vi "PID Template Multi-Channel PID.vi"(0 "process variable":i16, 1 "reset?":bool, 12 "configuration":T1) -> (4 "output":i16, 10 "channel index":u16)   [LabVIEW 2017]
uses:
  <vilib>/Platform/TimedLoop/XDataNode/timing_clust.ctl
  <vilib>/Platform/TimedLoop/XDataNode/nitl_modes.ctl
  <vilib>/Platform/TimedLoop/XDataNode/wakeup.ctl
  <vilib>/rvi/DataTransferAndStorage/Container/Common/niFpgaContainerGetUniqueNameForEmu.vi
  <vilib>/rvi/DataTransferAndStorage/Container/Common/niFpgaContainerSetEmuInfo.vi
  <vilib>/rvi/eio/common/nirviEmuReportErrorAndStop.vi
  <vilib>/Platform/TimedLoop/XDataNode/XDataNode.xnode
  <vilib>/rvi/LocalResourceManager/LocalResourceManager.xnode
  <vilib>/Platform/TimedLoop/XDataNode/XDNodeRunTimeDep.lvlib
  <vilib>/addons/control/pid/NI_PID_FPGA.lvlib
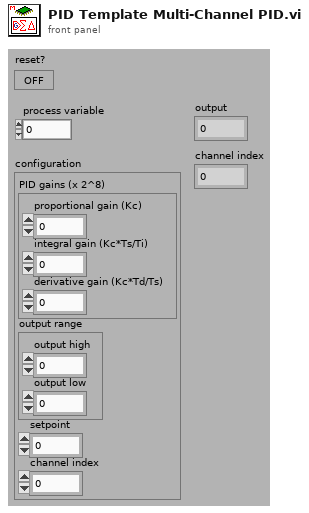
[diagram p1: front panel]
types:
  T1 = cluster{"PID gains (x 2^8)":cluster{"proportional gain (Kc)":i16, "integral gain (Kc*Ts/Ti)":i16, "derivative gain (Kc*Td/Ts)":i16}, "output range":cluster{"output high":i16, "output low":i16}, "setpoint":i16, "channel index":u16}
  T2 = typedef "XDNodeRunTimeDep.lvlib/timing_clust.ctl" = cluster{"Expected End [f-1]":u64, "Actual End [f-1]":u64, "Finished Late? [f-1]":bool, "Expected End [i-1]":u64, "Actual End [i-1]":u64, "Finished Late? [i-1]":bool, "Expected Start [i]":u64, "Actual Start [i]":u64, "Expected Start [f]":u64, "Actual Start [f]":u64, "Source Name":string, "Structure Name":string, "Period":i64, "Deadline":i64, "Offset":i64, "Start":i64, "Priority":i32, "Timeout":i32, "Mode":T3, "Wakeup Reason":T4, "Error":errorcluster, "Source Type":string, "Secondary Source Type":string, "Global End Time":u64, "Global Start Time":u64, "Frame Duration":u64, "Iteration Duration":u64, "Assigned CPU":i32, "I/O Scan Engine Mode":u32}
  T3 = typedef "XDNodeRunTimeDep.lvlib/nitl_modes.ctl" = enum32{"No Change", "Process missed periods, maintain original phase", "Discard missed periods, maintain original phase", "Process missed periods, ignore original phase", "Discard missed periods, ignore original phase"}
  T4 = typedef "XDNodeRunTimeDep.lvlib/wakeup.ctl" = enum32{"Normal", "Aborted", "Asynchronous wakeup", "Timing source error", "Timed loop error", "Timeout"}
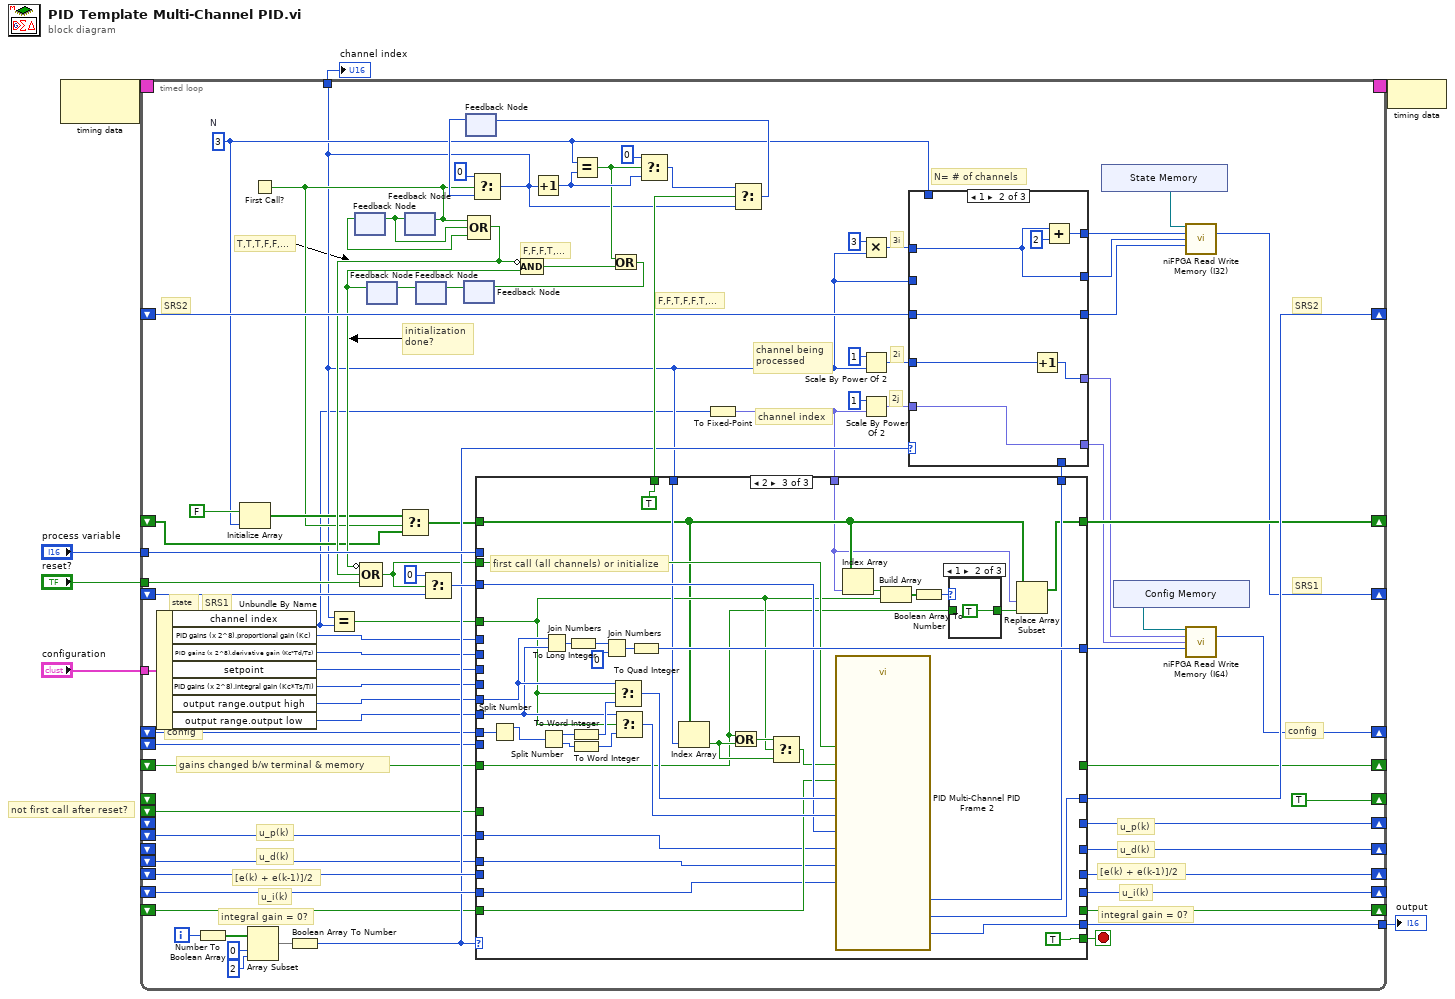
[diagram p0: block diagram]
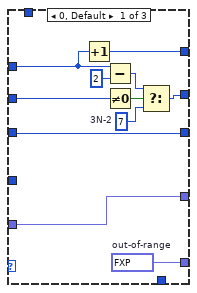
[diagram p2: hidden frame]
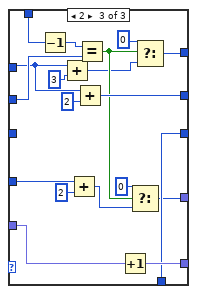
[diagram p3: hidden frame]
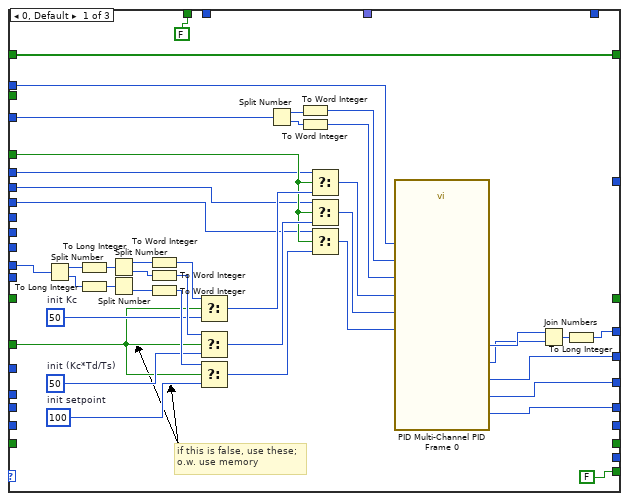
[diagram p4: hidden frame]
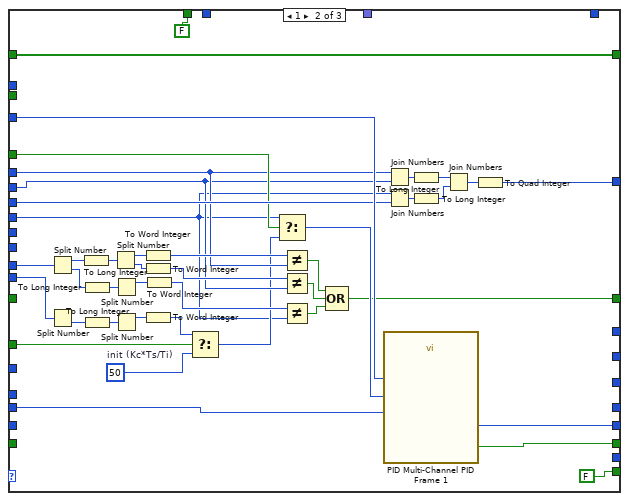
[diagram p5: hidden frame]
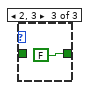
[diagram p7: hidden frame]
diagram:
  # "not first call after reset?"
  n1 = node-c288() -> (w7:T2)  [unwired: 1 out]
  n2 = timed-loop {
    timing: w7 -> [_]
    timing-out: [_] -> w6
    shift-right: [w89] -> _
    shift-left: _ -> [_]
    shift-right: [w90] -> _
    shift-left: _ -> [_]
    shift-right: [w88] -> _
    shift-left: _ -> [w58]
    tunnel: "process variable" -> [w87]
    shift-right: [w13] -> _
    shift-left: _ -> [w73]
    tunnel: "reset?" -> [w40]
    shift-right: [w80] -> _
    shift-left: _ -> [w79]
    shift-right: [w78] -> _
    shift-left: _ -> [w77]
    shift-right: [TRUE] -> _
    shift-right: [w12] -> _
    shift-left: _ -> [w59]
    shift-right: [w56] -> _
    shift-left: _ -> [w57]
    shift-left: _ -> [w60]
    shift-right: [w36] -> _
    shift-left: _ -> [w33]
    shift-left: _ -> [w47]
    shift-left: _ -> [w54]
    shift-left: _ -> [w53]
    shift-left: _ -> [_]
    tunnel: "configuration" -> [w39]
    tunnel: [w21] -> w2
    tunnel: [w37] -> w1
    shift-right: [w35] -> _
    shift-left: _ -> [w31]
    i -> [w71]
    stop <- w55 stop-if-true
    w28 = u16 3  # N
    # "2j"
    # "2i"
    # "3i"
    # "N= # of channels"
    # "F,F,T,F,F,T,..."
    # "F,F,F,T,..."
    # "T,T,T,F,F,..."
    # "config"
    # "channel index"
    # "channel being\nprocessed"
    # "SRS1"
    # "SRS2"
    # "SRS1"
    # "SRS2"
    # "config"
    # "state"
    # "u_i(k)"
    # "u_i(k)"
    # "initialization \ndone?"
    # "[e(k) + e(k-1)]/2"
    # "integral gain = 0?"
    # "u_d(k)"
    # "u_p(k)"
    # "[e(k) + e(k-1)]/2"
    # "u_p(k)"
    # "u_d(k)"
    # "integral gain = 0?"
    # "gains changed b/w terminal & memory"
    n3 = Unbundle By Name(w39) -> ("channel index"=w19:u16, "PID gains (x 2^8).proportional gain (Kc)"=w66:i16, "PID gains (x 2^8).derivative gain (Kc*Td/Ts)"=w65:i16, "setpoint"=w64:i16, "PID gains (x 2^8).integral gain (Kc*Ts/Ti)"=w63:i16, "output range.output high"=w62:i16, "output range.output low"=w61:i16)
    n4 = Number To Boolean Array(number=w71) -> (Boolean array=w76:bool[])
    n5 = Initialize Array(FALSE, w28) -> (w32:bool[])
    n6 = Array Subset(array=w76, index=0, length=2) -> (w72:bool[])
    n7 = First Call?() -> (First Call?: T/F=w29:bool)
    n8 = Boolean Array To Number(Boolean array=w72) -> (number=w68:u8)
    n9 = feedback #1() -> (w49:bool)  [unwired: 1 out]
    n10 = feedback #2() -> (w44:bool)  [unwired: 1 out]
    n11 = Select(t=w32, s=w29, f=w31) -> (s? t:f=w30:bool[])
    n12 = feedback-in #3(w29) -> ()
    n13 = feedback #3() -> (w50:bool)  [unwired: 1 out]
    n14 = feedback-in #1(w50) -> ()
    n15 = feedback #4() -> (w45:bool)  [unwired: 1 out]
    n16 = feedback-in #2(w45) -> ()
    n17 = feedback #5() -> (w43:bool)  [unwired: 1 out]
    n18 = feedback-in #4(w43) -> ()
    n19 = feedback #6() -> (w51:u16)  [unwired: 1 out]
    n20 = Compound Arithmetic op=OR(w29, w50, w49) -> (w48:bool)
    n21 = Compound Arithmetic op=OR(invert w44, w48, w40) -> (w41:bool)
    n22 = Select(t=0 ("Data"), s=w41, f=w73) -> (s? t:f=w69:i32)
    n23 = Select(t=u16 0, s=w29, f=w51) -> (s? t:f=w21:u16)
    n24 = Equal?(x=w21, y=w19) -> (x = y?=w67:bool)
    n25 = Compound Arithmetic op=AND(invert w48, w44) -> (w83:bool)
    n26 = Increment(x=w21) -> (x+1=w84:u16)
    n27 = Equal?(x=w28, y=w84) -> (x = y?=w82:bool)
    n28 = Or(x=w82, y=w83) -> (x .or. y?=w42:bool)
    n29 = feedback-in #5(w42) -> ()
    n30 = Select(t=u16 0, s=w82, f=w84) -> (s? t:f=w85:u16)
    n31 = To Fixed-Point(number=w19) -> (fixed-point=w18:fxp<+,17,17>)  [unwired: 1 out]
    n32 = case shown="2" w68 {
      tunnel: [w166 _ _] -> w90
      tunnel: [w167 _ _] -> w89
      tunnel: [_ w209 _] -> w88
      tunnel: w54 -> [_ _ w213]
      tunnel: w53 -> [_ _ w212]
      tunnel: w87 -> [w164 _ _]
      tunnel: [FALSE FALSE TRUE] -> w81
      tunnel: [w165 _ _] -> w80
      tunnel: w79 -> [_ w184 _]
      tunnel: [_ w208 _] -> w78
      tunnel: w77 -> [_ _ w211]
      tunnel: w69 -> [w161 w207 w236]
      tunnel: [w157 _ w233] -> w56
      tunnel: [_ w175 _] -> w36
      tunnel: w67 -> [w135 w176 w221]
      tunnel: w66 -> [w134 w174 _]
      tunnel: w65 -> [w133 w173 _]
      tunnel: w64 -> [w132 w183 _]
      tunnel: w63 -> [_ w170 _]
      tunnel: w62 -> [_ _ w238]
      tunnel: w61 -> [_ _ w237]
      tunnel: w60 -> [_ w186 _]
      tunnel: w47 -> [w137 w188 _]
      tunnel: w59 -> [w136 w189 w247]
      tunnel: [_ w179 w240] -> w9
      tunnel: w58 -> [_ _ w232]
      tunnel: w33 -> [_ _ w215]
      tunnel: [FALSE FALSE TRUE] -> w55
      tunnel: w41 -> [_ _ w229]
      tunnel: [_ _ w231] -> w38
      tunnel: [_ _ w230] -> w37
      tunnel: w30 -> [w128 w169 w218]
      tunnel: w21 -> [_ _ w226]
      tunnel: w18 -> [_ _ w217]
      tunnel: [w128 w169 w225] -> w35
      frame 0, Default {
        w141 = i16 100  # init setpoint
        w143 = i16 50  # init Kc
        w142 = i16 50  # init (Kc*Td/Ts)
        # "if this is false, use these; \no.w. use memory"
        n33 = Split Number(x=w136) -> (hi(x)=w144:u32, lo(x)=w145:u32)
        n34 = To Long Integer(number=w144) -> (32bit integer=w155:i32)
        n35 = To Long Integer(number=w145) -> (32bit integer=w156:i32)
        n36 = Split Number(x=w155) -> (hi(x)=w146:u16, lo(x)=w148:u16)
        n37 = Split Number(x=w156) -> (lo(x)=w150:u16)  [unwired: 1 out]
        n38 = To Word Integer(number=w146) -> (16bit integer=w147:i16)
        n39 = To Word Integer(number=w148) -> (16bit integer=w149:i16)
        n40 = To Word Integer(number=w150) -> (16bit integer=w151:i16)
        n41 = Select(t=w147, s=w137, f=w143) -> (s? t:f=w152:i16)
        n42 = Select(t=w149, s=w137, f=w142) -> (s? t:f=w153:i16)
        n43 = Select(t=w151, s=w137, f=w141) -> (s? t:f=w154:i16)
        n44 = Split Number(x=w161) -> (hi(x)=w162:u16, lo(x)=w163:u16)
        n45 = To Word Integer(number=w162) -> (16bit integer=w160:i16)
        n46 = To Word Integer(number=w163) -> (16bit integer=w159:i16)
        n47 = Select(t=w134, s=w135, f=w152) -> (s? t:f=w140:i16)
        n48 = Select(t=w133, s=w135, f=w153) -> (s? t:f=w139:i16)
        n49 = Select(t=w132, s=w135, f=w154) -> (s? t:f=w138:i16)
        n50 = call <vilib>:"PID Multi-Channel PID Frame 0.vi"("setpoint"=w138, "proportional gain (Kc) (k)"=w140, "derivative gain (Kc*Td/Ts) (k)"=w139, "PV(k)"=w164, "e(k-1)"=w159, "PV(k-1)"=w160) -> ("[e(k)+e(k-1)]/2"=w165:i16, "PV(k)"=w131:i16, "e(k)"=w130:i16, "u_p(k)"=w167:i32, "u_d(k)"=w166:i32)  [unwired: 5 out]
        n51 = Join Numbers(hi=w131, lo=w130) -> ((hi.lo)=w158:u32)
        n52 = To Long Integer(number=w158) -> (32bit integer=w157:i32)
      }
      frame 1 {
        w187 = i16 50  # init (Kc*Ts/Ti)
        n53 = Split Number(x=w189) -> (hi(x)=w194:u32, lo(x)=w198:u32)
        n54 = Split Number(x=w186) -> (lo(x)=w191:u32)  [unwired: 1 out]
        n55 = To Long Integer(number=w194) -> (32bit integer=w195:i32)
        n56 = To Long Integer(number=w198) -> (32bit integer=w197:i32)
        n57 = To Long Integer(number=w191) -> (32bit integer=w192:i32)
        n58 = Split Number(x=w195) -> (hi(x)=w196:u16, lo(x)=w199:u16)
        n59 = Split Number(x=w197) -> (hi(x)=w200:u16)  [unwired: 1 out]
        n60 = Split Number(x=w192) -> (hi(x)=w193:u16)  [unwired: 1 out]
        n61 = To Word Integer(number=w196) -> (16bit integer=w201:i16)
        n62 = To Word Integer(number=w199) -> (16bit integer=w202:i16)
        n63 = To Word Integer(number=w193) -> (16bit integer=w185:i16)
        n64 = To Word Integer(number=w200) -> (16bit integer=w203:i16)
        n65 = Select(t=w185, s=w188, f=w187) -> (s? t:f=w172:i16)
        n66 = Select(t=w170, s=w176, f=w172) -> (s? t:f=w190:i16)
        n67 = Not Equal?(x=w201, y=w174) -> (x != y?=w204:bool)
        n68 = Not Equal?(x=w202, y=w173) -> (x != y?=w205:bool)
        n69 = Not Equal?(x=w203, y=w170) -> (x != y?=w206:bool)
        n70 = Compound Arithmetic op=OR(w204, w205, w206) -> (w175:bool)
        n71 = call <vilib>:"PID Multi-Channel PID Frame 1.vi"("ie(k-1)"=w207, "integral gain (Kc*Ts/Ti) (k)"=w190, "[e(k)+e(k-1)]/2"=w184) -> ("u_i(k)"=w208:i32, "integration off"=w209:bool)  [unwired: 11 out]
        n72 = Join Numbers(hi=w174, lo=w173) -> ((hi.lo)=w182:u32)
        n73 = Join Numbers(hi=w170, lo=w183) -> ((hi.lo)=w181:u32)
        n74 = To Long Integer(number=w182) -> (32bit integer=w178:i32)
        n75 = To Long Integer(number=w181) -> (32bit integer=w177:i32)
        n76 = Join Numbers(hi=w178, lo=w177) -> ((hi.lo)=w180:u64)
        n77 = To Quad Integer(1:w180) -> (0:w179:i64)
      }
      frame 2 {
        # "first call (all channels) or initialize"
        n78 = Split Number(x=w247) -> (hi(x)=w235:u32)  [unwired: 1 out]
        n79 = Split Number(x=w235) -> (hi(x)=w248:u16, lo(x)=w228:u16)
        n80 = Join Numbers(hi=w238, lo=w237) -> ((hi.lo)=w242:u32)
        n81 = To Long Integer(number=w242) -> (32bit integer=w241:i32)
        n82 = To Word Integer(number=w248) -> (16bit integer=w244:i16)
        n83 = To Word Integer(number=w228) -> (16bit integer=w243:i16)
        n84 = Join Numbers(hi=w241, lo=0) -> ((hi.lo)=w239:u64)
        n85 = Select(t=w238, s=w221, f=w244) -> (s? t:f=w245:i16)
        n86 = Select(t=w237, s=w221, f=w243) -> (s? t:f=w246:i16)
        n87 = To Quad Integer(1:w239) -> (0:w240:i64)
        n88 = Index Array(array=w218, index=w226) -> (element=w224:bool)
        n89 = Or(x=w215, y=w224) -> (x .or. y?=w223:bool)
        n90 = Select(t=w223, s=w221, f=w224) -> (s? t:f=w222:bool)
        n91 = call <vilib>:"PID Multi-Channel PID Frame 2.vi"("output(k-1)"=w236, "output range high"=w245, "output range low"=w246, "u_p(k)"=w213, "u_i(k)"=w211, "u_d(k)"=w212, "first call or initialize?"=w229, "integration off?"=w232, "gains changed?"=w222) -> ("output"=w230:i16, "integrated effort(k)"=w233:i32, "unscaled output(k)"=w231:i32)  [unwired: 4 out]
        n92 = Index Array(array=w218, index=w217) -> (element=w214:bool)
        n93 = Build Array(w214, w221) -> (w220:bool[])
        n94 = Boolean Array To Number(Boolean array=w220) -> (number=w219:u8)
        n95 = case shown="1" w219 {
          tunnel: [w250 TRUE FALSE] -> w216
          tunnel: w215 -> [w250 _ _]
          frame 0, Default {
          }
          frame 1 {
          }
          frame 2, 3 {
          }
        }
        n96 = Replace Array Subset(array=w218, new element=w216, index=w217) -> (w225:bool[])
      }
    }
    n97 = Select(t=w85, s=w81, f=w21) -> (s? t:f=w52:u16)
    n98 = feedback-in #6(w52) -> ()
    n99 = Multiply(x=u16 3 ("Data"), y=w21) -> (x*y=w26:u16)
    n100 = Scale By Power Of 2(n=u16 1 ("Data"), x=w21) -> (x*2^n=w22:u16)
    n101 = Scale By Power Of 2(n=u16 1 ("Data"), x=w18) -> (x*2^n=w24:fxp<+,17,17>)
    n102 = case shown="1" w68 {
      tunnel: [w93 w108 w120] -> w10
      tunnel: w21 -> [w96 _ w118]
      tunnel: [w91 w102 w127] -> w8
      tunnel: [w101 w106 w124] -> w16
      tunnel: [w100 w105 w125] -> w14
      tunnel: w57 -> [w100 w105 _]
      tunnel: [w98 w104 w126] -> w15
      tunnel: w38 -> [_ _ w125]
      tunnel: w28 -> [_ _ w117]
      tunnel: w26 -> [w94 w104 w114]
      tunnel: w24 -> [w93 w102 w109]
      tunnel: w22 -> [_ w103 w111]
      frame 0, Default {
        w91 = fxp<+,18,18> 131072.0  # out-of-range
        w92 = u16 7  # 3N-2
        n103 = Increment(x=w94) -> (x+1=w101:u16)
        n104 = Subtract(x=w94, y=u16 2 ("Data")) -> (x-y=w95:u16)
        n105 = Not Equal To 0?(x=w96) -> (x != 0?=w97:bool)
        n106 = Select(t=w95, s=w97, f=w92) -> (s? t:f=w98:u16)
      }
      frame 1 {
        n107 = Increment(x=w103) -> (x+1=w108:u16)
        n108 = Add(x=w104, y=u16 2 ("Data")) -> (x+y=w106:u16)
      }
      frame 2 {
        n109 = Decrement(x=w117) -> (x-1=w123:u16)
        n110 = Add(x=w114, y=u16 3 ("Data")) -> (x+y=w115:u16)
        n111 = Add(x=w111, y=u16 2 ("Data")) -> (x+y=w110:u16)
        n112 = Add(x=w114, y=u16 2 ("Data")) -> (x+y=w126:u16)
        n113 = Equal?(x=w123, y=w118) -> (x = y?=w121:bool)
        n114 = Increment(x=w109) -> (x+1=w127:fxp<+,18,18>)
        n115 = Select(t=u16 0 ("Data"), s=w121, f=w110) -> (s? t:f=w120:u16)
        n116 = Select(t=u16 0 ("Data"), s=w121, f=w115) -> (s? t:f=w124:u16)
      }
    }
    n117 = xnode ("State Memory")() -> ("Memory Out"=w17:refnum<k21>)
    n118 = xnode ("Config Memory")() -> ("Memory Out"=w11:refnum<k21>)
    n119 = call <vilib>:"niFPGA Read Write Memory (I32).vi"("memory"=w17, "read address"=w16, "write address"=w15, "data in"=w14) -> ("data out"=w13:i32)  [unwired: 11 in]
    n120 = call <vilib>:"niFPGA Read Write Memory (I64).vi"("memory"=w11, "read address"=w10, "write address"=w8, "data in"=w9) -> ("data out"=w12:i64)  [unwired: 11 in]
  }
  "channel index" <- w2
  "output" <- w1
  n121 = node-c288(w6) -> ()
